vi "forcedDraftInd.vi"(8 "error in":errorcluster, 9 "Boiler Simulation Controls":refnum<vi>, 10 "Boiler Controls":refnum<vi>, 11 "Boiler Status Indicators":refnum<vi>) -> (0 "error out":errorcluster)   [LabVIEW 2024]
uses:
  Controls/Boiler Simulation Controls.ctl
  Controls/Boiler Status Indicators.ctl
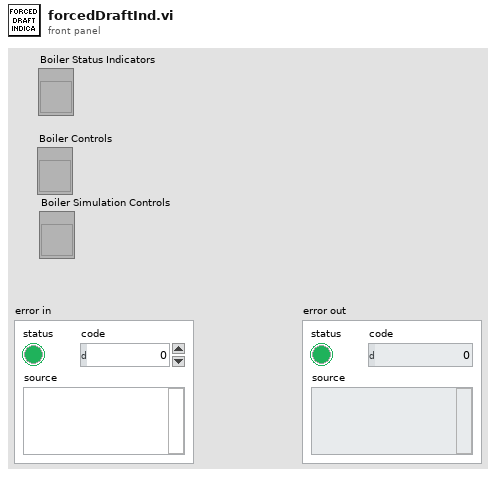
[diagram p1: front panel]
types:
  T1 = typedef "Boiler Simulation Controls.ctl" = cluster{"Flame Sensor Value (%)":dbl, "Run Interlock":bool, "Forced Draft Fan":bool}
  T2 = typedef "Boiler Status Indicators.ctl" = cluster{"Status":string, "Primary Fan":bool, "Natural Gas Valve":bool, "Pilot":bool, "Fuel Valve":bool, "Forced Draft Fan":bool, "Time Count":dbl}
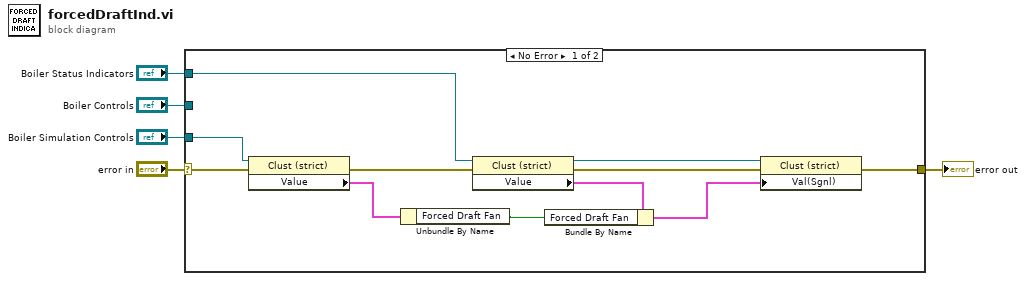
[diagram p0: block diagram]
diagram:
  n1 = case shown="No Error" "error in" {
    selector: "error in" -> [w10 w17]
    tunnel: [w12 w17] -> w4
    tunnel: "Boiler Status Indicators" -> [w11 _]
    tunnel: "Boiler Controls" -> [_ _]
    tunnel: "Boiler Simulation Controls" -> [w8 _]
    frame No Error {
      n2 = property class="Clust (strict)"(reference=w8, error in=w10) -> (error out=w9:errorcluster, "Value"=w7:T1)  [unwired: 1 out]
      n3 = Unbundle By Name(w7) -> ("Forced Draft Fan"=w6:bool)
      n4 = property class="Clust (strict)"(reference=w11, error in=w9) -> (reference out=w14:refnum<vi>, error out=w13:errorcluster, "Value"=w16:T2)
      n5 = Bundle By Name(cluster=w16, "Forced Draft Fan"=w6) -> (w15:T2)
      n6 = property class="Clust (strict)"(reference=w14, error in=w13, "Val(Sgnl)"=w15) -> (error out=w12:errorcluster)  [unwired: 1 out]
    }
    frame Error {
    }
  }
  "error out" <- w4
